vi "FilterMetrics.vi"(11 "supported metrics":string[](array[string])) -> (2 "low rate supported metrics":string[](array[string]), 3 "high rate supported metrics":string[](array[string]))   [LabVIEW 2017, in "CmsAnalysis.lvlib"]
uses:
  <vilib>/addons/InsightCM/Devices/Shared/Cms/CmsAnalysis/CmsAnalysis.lvlib
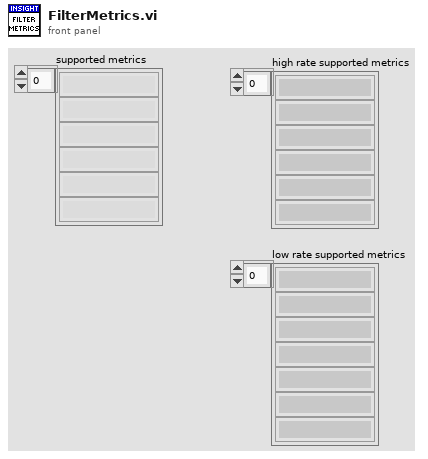
[diagram p1: front panel]
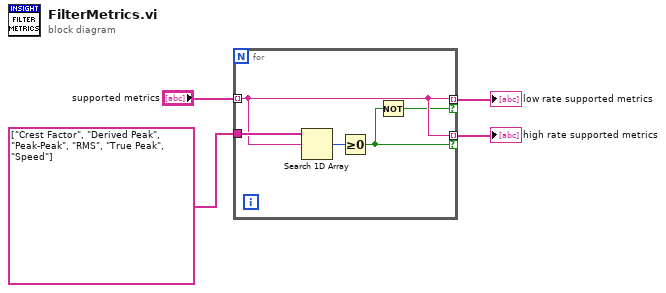
[diagram p0: block diagram]
diagram:
  n1 = for {
    tunnel: "supported metrics" -> [w7] mode=indexing
    tunnel: string[] ["Crest Factor", "Derived Peak", "Peak-Peak", "RMS", "True Peak", "Speed"] ("value") -> [w9]
    tunnel: [w7] -> w2 mode=indexing if=w5
    tunnel: [w7] -> w1 mode=indexing if=w6
    n2 = Search 1D Array(1D array=w9, element=w7) -> (index of element=w8:i32)  [unwired: 1 in]
    n3 = Greater Or Equal To 0?(x=w8) -> (x >= 0?=w5:bool)
    n4 = Not(x=w5) -> (.not. x?=w6:bool)
  }
  "high rate supported metrics" <- w2
  "low rate supported metrics" <- w1
